vi "ReadStimulusGivenCameraFrame.vi"(8 "error in (no error)":errorcluster, 10 "CameraFrame":i32, 11 "StimulusObject in":refnum<class "StimulusObject.lvclass">) -> (0 "error out":errorcluster, 2 "StimulusForFrame":sgl[](array[numeric]), 3 "StimulusObject out":refnum<class "StimulusObject.lvclass">)   [LabVIEW 2019, in "StimulusObject.lvclass"]
uses:
  StimulusObject.lvclass
  StimulusObject.lvclass/StimulusObject.ctl
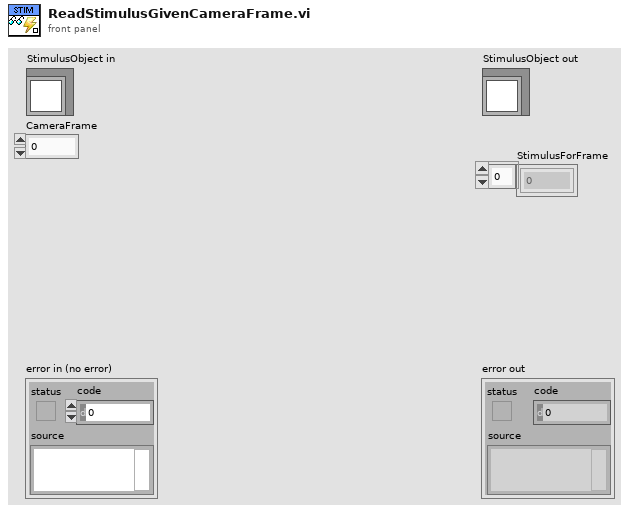
[diagram p1: front panel]
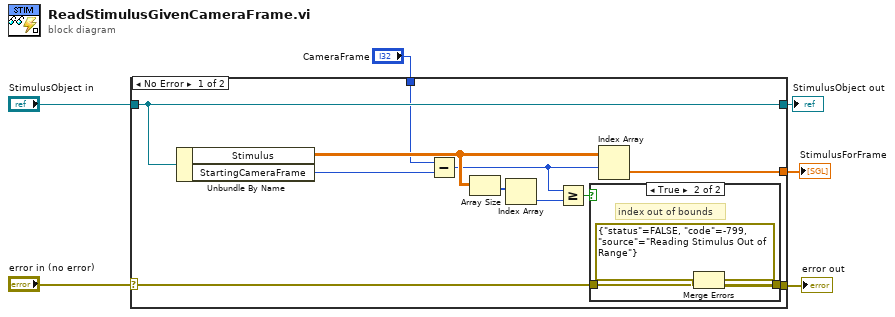
[diagram p0: block diagram]
diagram:
  n1 = case shown="No Error" "error in (no error)" {
    selector: "error in (no error)" -> [w10 w22]
    tunnel: [w9 w22] -> w5
    tunnel: [w17 w23] -> w3
    tunnel: "StimulusObject in" -> [w17 w23]
    tunnel: [w16 _] -> w2
    tunnel: "CameraFrame" -> [w7 _]
    frame No Error {
      n2 = Unbundle By Name(w17) -> ("Stimulus"=w14:sgl[][], "StartingCameraFrame"=w15:i32)
      n3 = Subtract(x=w7, y=w15) -> (x-y=w12:i32)
      n4 = Array Size(array=w14) -> (size(s)=w13:i32[])
      n5 = Index Array(array=w13) -> (element=w11:i32)  [unwired: 1 in]
      n6 = Greater Or Equal?(x=w12, y=w11) -> (x >= y?=w8:bool)
      n7 = case shown="True" w8 {
        tunnel: w10 -> [w18 w20]
        tunnel: [w18 w21] -> w9
        frame False {
        }
        frame True {
          # "index out of bounds"
          n8 = Merge Errors(errorcluster {"status"=FALSE, "code"=-799, "source"="Reading Stimulus Out of Range"} ("error IO"), w20) -> (w21:errorcluster)
        }
      }
      n9 = Index Array(array=w14, index (row)=w12) -> (element=w16:sgl[])  [unwired: 1 in]
    }
    frame Error {
    }
  }
  "error out" <- w5
  "StimulusObject out" <- w3
  "StimulusForFrame" <- w2
